vi "Global variable.vi"() -> ()   [LabVIEW 2019]
panel:
  in  "图数据":dbl[][](array[numeric])
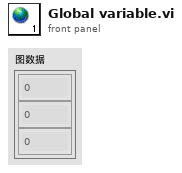
[diagram p1: front panel]
diagram:
